vi "Update Methods Event Structures.vi"(8 "error in (no error)":errorcluster, 10 "RPC Method Parameters":T1, 11 "LVClassLibrary in":refnum<vi>) -> (0 "error out":errorcluster, 3 "LVClassLibrary out":refnum<vi>)   [LabVIEW 2019, in "gRPC Template Creation Utility.lvlib"]
uses:
  gRPC Template Creation Utility.lvlib
  TypeDefs/RPC Method Parameters.ctl
  <vilib>/event_ctls.llb/lveventtype.ctl
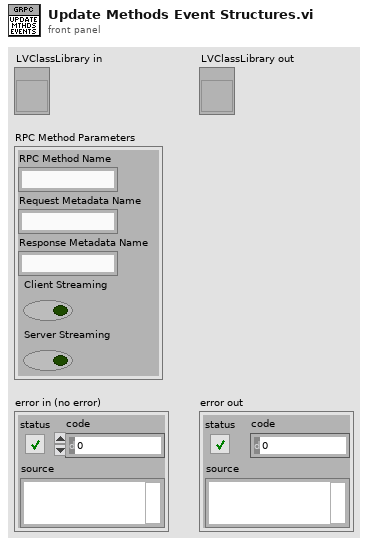
[diagram p1: front panel]
types:
  T1 = typedef "gRPC Template Creation Utility.lvlib/RPC Method Parameters.ctl" = cluster{"RPC Method Name":string, "Request Metadata Name":string, "Response Metadata Name":string, "Client Streaming":bool, "Server Streaming":bool}
  T2 = typedef "lveventtype.ctl" = enum32{"Null", "Timeout", "Annotation Menu Selection", "Annotation Menu Selection?", "App Instance Close", "App Instance Close?", "Autoscale Range Change", "Bookmark Info Change", "Cell Edit", "Cell Edit?", "Cursor Grab", "Cursor Grab?", "Cursor Menu Selection", "Cursor Menu Selection?", "Cursor Move", "Cursor Release", "Data Change", "Direction Change", "Display State Change", "Drag Ended", "Drag Enter", "Drag Leave", "Drag Over", "Drag Source Update", "Drag Starting", "Drag Starting?", "Drop", "Exec State Change", "Key Down", "Key Down?", "Key Repeat", "Key Repeat?", "Key Up", "Listbox Double Click", "Menu Activation?", "Menu Selection (App)", "Menu Selection? (App)", "Menu Selection (User)", "Mouse Down", "Mouse Down?", "Mouse Enter", "Mouse Leave", "Mouse Move", "Mouse Up", "Mouse Wheel", "NI Security User Change (App)", "Pane Size", "Panel Close", "Panel Close?", "Panel Resize", "Plot Attribute Change", "Scale Range Change", "Shortcut Menu Activation?", "Shortcut Menu Selection (App)", "Shortcut Menu Selection? (App)", "Shortcut Menu Selection (User)", "Tree Double Click", "Tree Drag", "Tree Drag?", "Tree Drop", "Tree Drop?", "Tree Item Close", "Tree Item Close?", "Tree Item Open", "Tree Item Open?", "User Event", "Value Change"}
  T3 = cluster{"Event Type":T2, "Event Registration Index":i32}[]
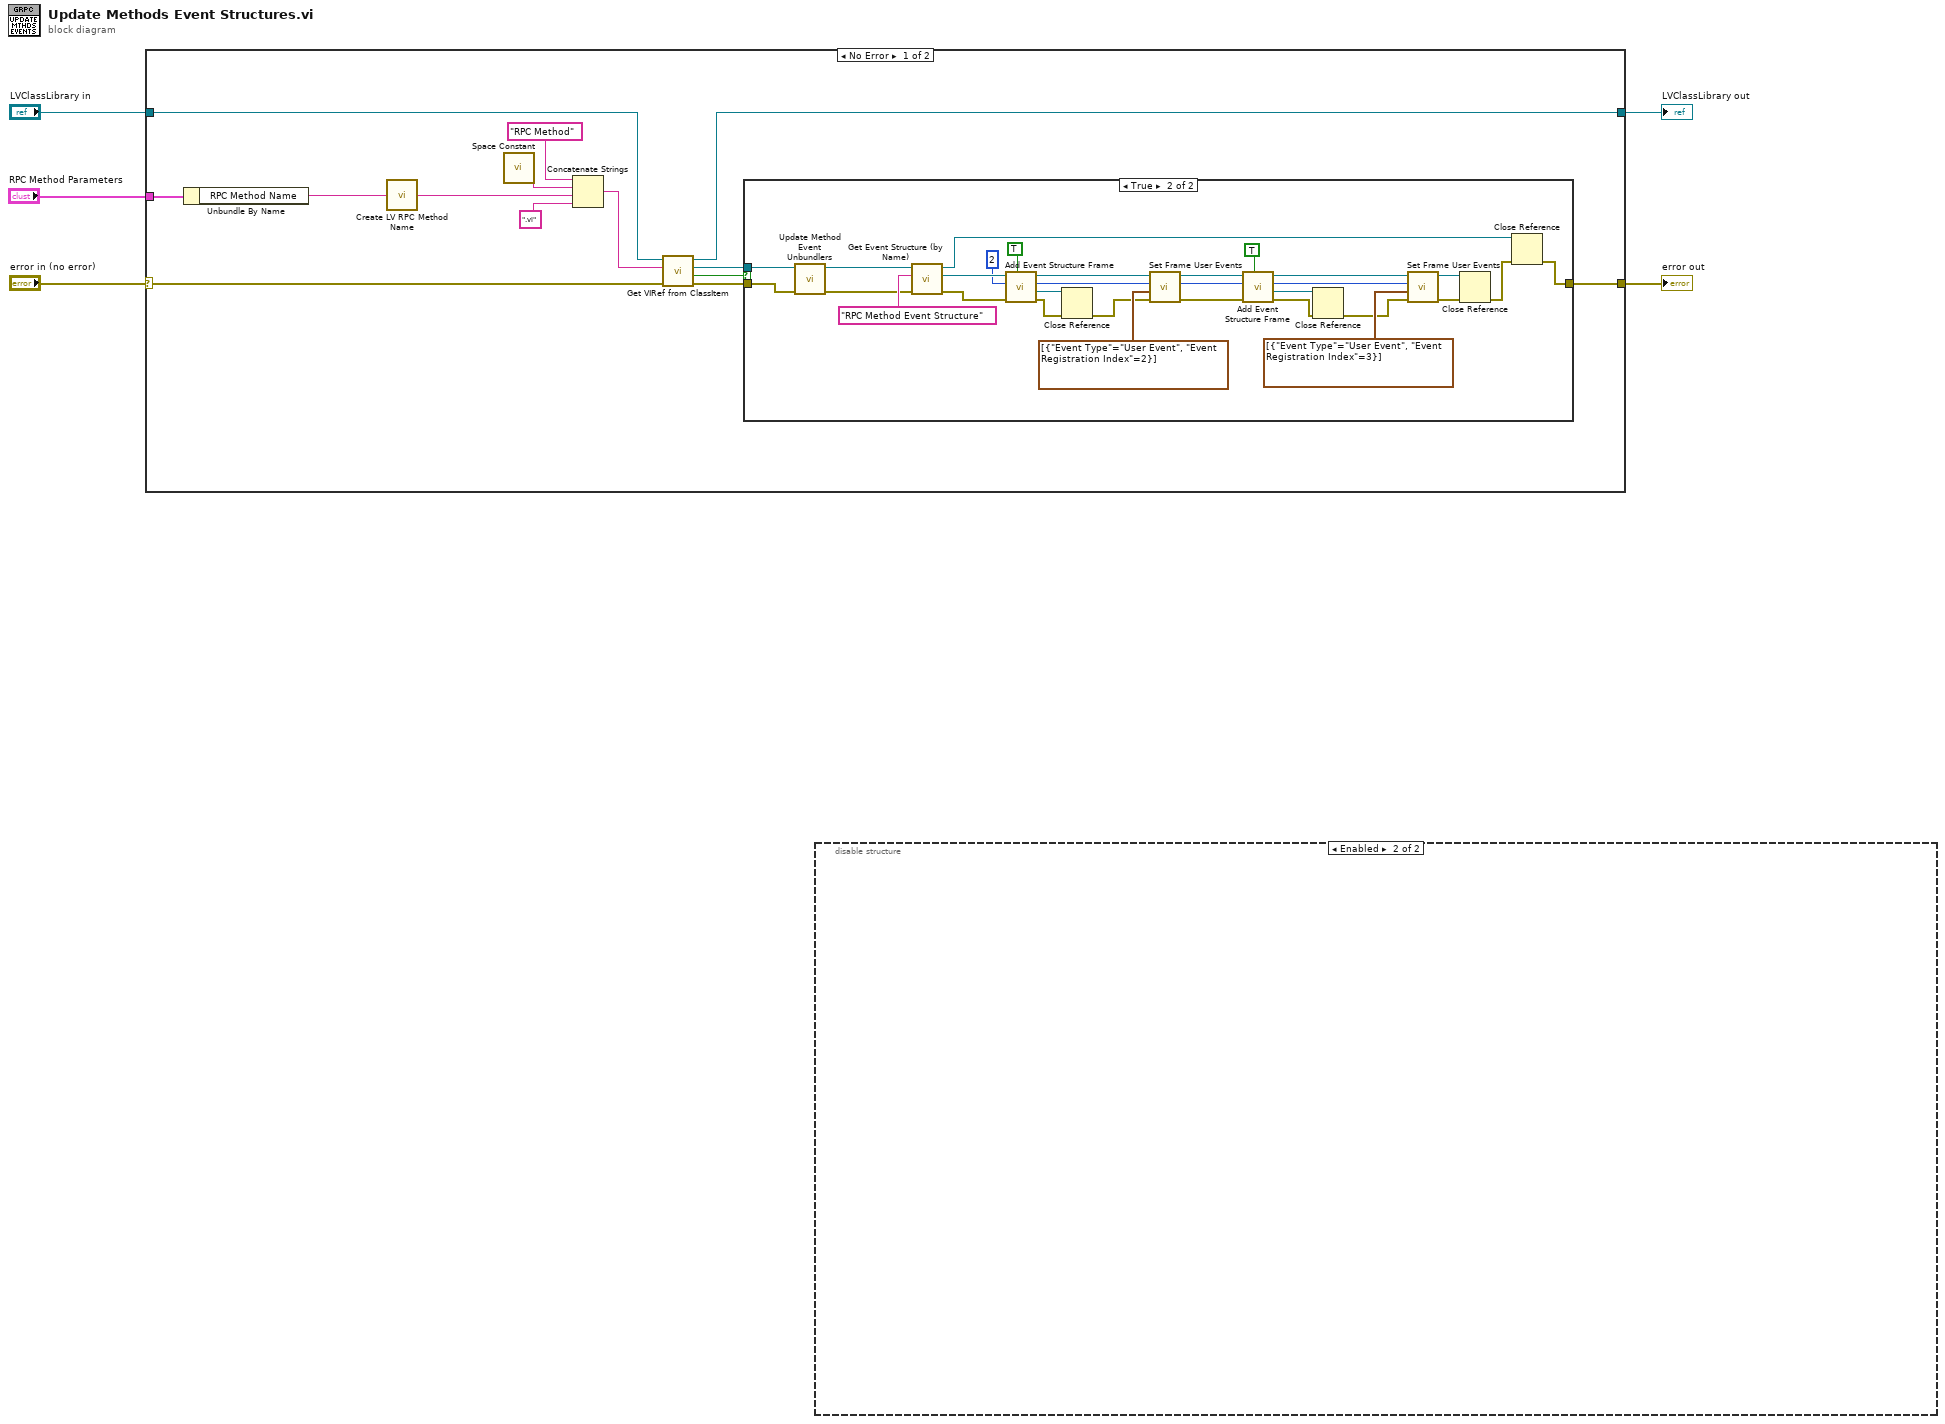
[diagram p0: block diagram]
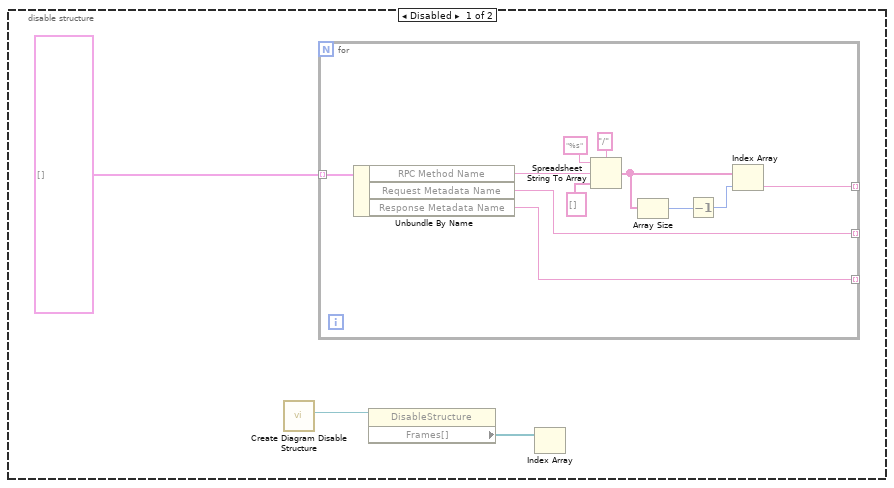
[diagram p4: hidden frame]
diagram:
  n1 = case shown="No Error" "error in (no error)" {
    selector: "error in (no error)" -> [w19 w52]
    tunnel: [w10 w51] -> w5
    tunnel: "LVClassLibrary in" -> [w14 w51]
    tunnel: [w9 w52] -> w3
    tunnel: "RPC Method Parameters" -> [w8 _]
    frame No Error {
      n2 = Unbundle By Name(w8) -> ("RPC Method Name"=w7:string)
      n3 = call "Create LV RPC Method Name.vi"("Proto Parser RPC Method Name in"=w7) -> ("LV RPC Method Name out"=w6:string)
      n4 = call <vilib>:"Space Constant.vi"() -> ("String"=w17:string)
      n5 = Concatenate Strings("RPC Method" ("regular expression"), w17, w6, ".vi" ("string")) -> (w15:string)
      n6 = call "Get VIRef from ClassItem.vi"("error in (no error)"=w19, "Item Name"=w15, "LVClassLibrary in"=w14) -> ("error out"=w13:errorcluster, "Found ?"=w11:bool, "VIref out"=w12:refnum<vi>, "LVClassLibrary out"=w10:refnum<vi>)  [unwired: 5 in]
      n7 = case shown="True" w11 {
        tunnel: [w20 w50] -> w9
        tunnel: w13 -> [w20 w22]
        tunnel: w12 -> [_ w21]
        frame False {
        }
        frame True {
          n8 = call "Update Method Event Unbundlers.vi"("error in (no error)"=w22, "VI ref in"=w21) -> ("error out"=w47:errorcluster, "VI ref out"=w49:refnum<vi>)  [unwired: 7 in, 1 out]
          n9 = call "Get Event Structure (by Name).vi"("error in (no error)"=w47, "Label"="RPC Method Event Structure", "Owner VI in"=w49) -> ("error out"=w45:errorcluster, "Event Structure ref out"=w46:refnum<vi>, "Owner VI out"=w27:refnum<vi>)  [unwired: 5 in, 1 out]
          n10 = call "Add Event Structure Frame.vi"("After? (T)"=TRUE, "error in (no error)"=w45, "Reference Frame Index"=u32 2, "Event Structure ref in"=w46) -> ("error out"=w23:errorcluster, "Added Frame"=w24:refnum<vi>, "Added Frame Index"=w41:i32, "Event Structure ref out"=w44:refnum<vi>)  [unwired: 4 in]
          n11 = Close Reference(reference=w24, error in (no error)=w23) -> (error out=w30:errorcluster)
          n12 = call "Set Frame User Events.vi"("error in (no error)"=w30, "Dynamic Events"=T3 [{"Event Type"=enum."User Event", "Event Registration Index"=2}], "Frame Index in"=w41, "Event Structure ref in"=w44) -> ("error out"=w36:errorcluster, "Frame Index out"=w34:i32, "Event Structure ref out"=w35:refnum<vi>)  [unwired: 5 in]
          n13 = call "Add Event Structure Frame.vi"("After? (T)"=TRUE, "error in (no error)"=w36, "Reference Frame Index"=w34, "Event Structure ref in"=w35) -> ("error out"=w25:errorcluster, "Added Frame"=w26:refnum<vi>, "Added Frame Index"=w38:i32, "Event Structure ref out"=w37:refnum<vi>)  [unwired: 4 in]
          n14 = Close Reference(reference=w26, error in (no error)=w25) -> (error out=w29:errorcluster)
          n15 = call "Set Frame User Events.vi"("error in (no error)"=w29, "Dynamic Events"=T3 [{"Event Type"=enum."User Event", "Event Registration Index"=3}], "Frame Index in"=w38, "Event Structure ref in"=w37) -> ("error out"=w32:errorcluster, "Event Structure ref out"=w31:refnum<vi>)  [unwired: 5 in, 1 out]
          n16 = Close Reference(reference=w31, error in (no error)=w32) -> (error out=w28:errorcluster)
          n17 = Close Reference(reference=w27, error in (no error)=w28) -> (error out=w50:errorcluster)
        }
      }
    }
    frame Error {
    }
  }
  "error out" <- w3
  "LVClassLibrary out" <- w5
  n18 = disable-structure shown="Enabled" {
    frame Disabled {
      n19 = call "Create Diagram Disable Structure.vi"() -> ("DDS  Ref out"=w53:refnum<vi>)  [unwired: 9 in, 2 out]
      n20 = for {
        tunnel: T1[] [] ("RPC Method Parameters") -> [w66] mode=indexing
        tunnel: [w58] -> _ mode=indexing
        tunnel: [w57] -> _ mode=indexing
        tunnel: [w56] -> _ mode=indexing
        n21 = Unbundle By Name(w66) -> ("RPC Method Name"=w59:string, "Request Metadata Name"=w57:string, "Response Metadata Name"=w56:string)
        n22 = Spreadsheet String To Array(delimiter (Tab)="/", format string="%s", spreadsheet string=w59, array type (2D Dbl)=string[] []) -> (array=w60:string[])
        n23 = Array Size(array=w60) -> (size(s)=w62:i32)
        n24 = Decrement(x=w62) -> (x-1=w61:i32)
        n25 = Index Array(array=w60, index=w61) -> (element=w58:string)
      }
      n26 = property class="DisableStructure"(reference=w53) -> ("Frames[]"=w54:refnum<vi>[])  [unwired: 1 in, 2 out]
      n27 = Index Array(array=w54) -> ()  [unwired: 1 in, 1 out]
    }
    frame Enabled {
    }
  }
